vi "Main_RT.vi"() -> ()   [LabVIEW 2015]
uses:
  <vilib>/NI/Software Watchdog/Pound/Pound.lvclass
  <vilib>/addons/InsightCM/Devices/Shared/AcquireScanEngine/ScanEngine.lvlib
  <vilib>/addons/InsightCM/Devices/Shared/VibrationAnalysisLoop/VibrationAnalysis.lvlib
  <vilib>/addons/InsightCM/Devices/Shared/Trigger/Trigger.lvlib
  <vilib>/addons/InsightCM/Devices/Shared/TdmsCreator/TdmsCreator.lvlib
  <vilib>/addons/TraceLogger/TraceLogger.lvlib
  <vilib>/addons/TimerProcess/TimerProcess.lvlib
  <vilib>/addons/BlinkProcess/BlinkProcess.lvlib
  <vilib>/addons/InsightCM/Devices/Shared/Controller/Controller.lvlib
  <vilib>/addons/InsightCM/Devices/Shared/ServerComm/ServerComm.lvlib
  <vilib>/addons/InsightCM/Devices/Shared/FileManager/FileManager.lvlib
  <vilib>/addons/InsightCM/Devices/Shared/TracePointDisplay/TracePointDisplay.lvlib
  <vilib>/addons/InsightCM/Devices/Shared/TagPublish/TagPublish.lvlib
  <vilib>/addons/InsightCM/Devices/Shared/DataAccumulatorProcess/DataAccumulator.lvlib
  <vilib>/addons/InsightCM/Devices/Shared/DeviceHealth/DeviceHealth.lvlib
  <vilib>/addons/InsightCM/Devices/Shared/SinglePointClock/SinglePointClock.lvlib
  <vilib>/addons/InsightCM/Devices/Shared/VibrationVirtualChannel/VibrationVirtualChannel.lvlib
  <vilib>/addons/InsightCM/Devices/Shared/Alarm/Alarm.lvlib
  <vilib>/addons/InsightCM/Devices/Shared/TestPanel/TestPanel.lvlib
  <vilib>/addons/InsightCM/Devices/Shared/DataExplorerHelper/DataExplorerHelper.lvlib
  <vilib>/addons/InsightCM/Devices/Shared/ModbusMaster/ModbusMaster.lvlib
  <vilib>/addons/WatchdogProcess/WatchdogProcess.lvlib
panel:
  out "debug":string
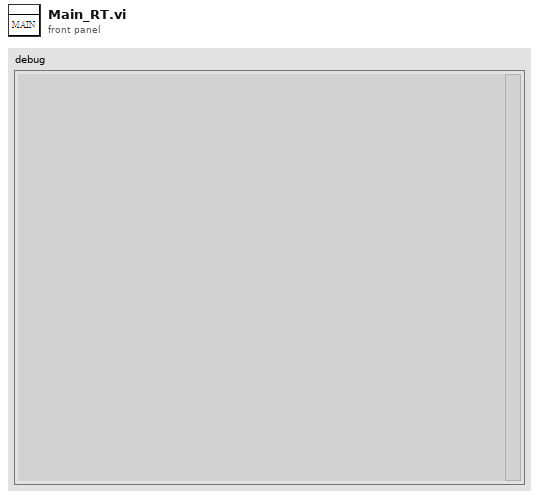
[diagram p1: front panel]
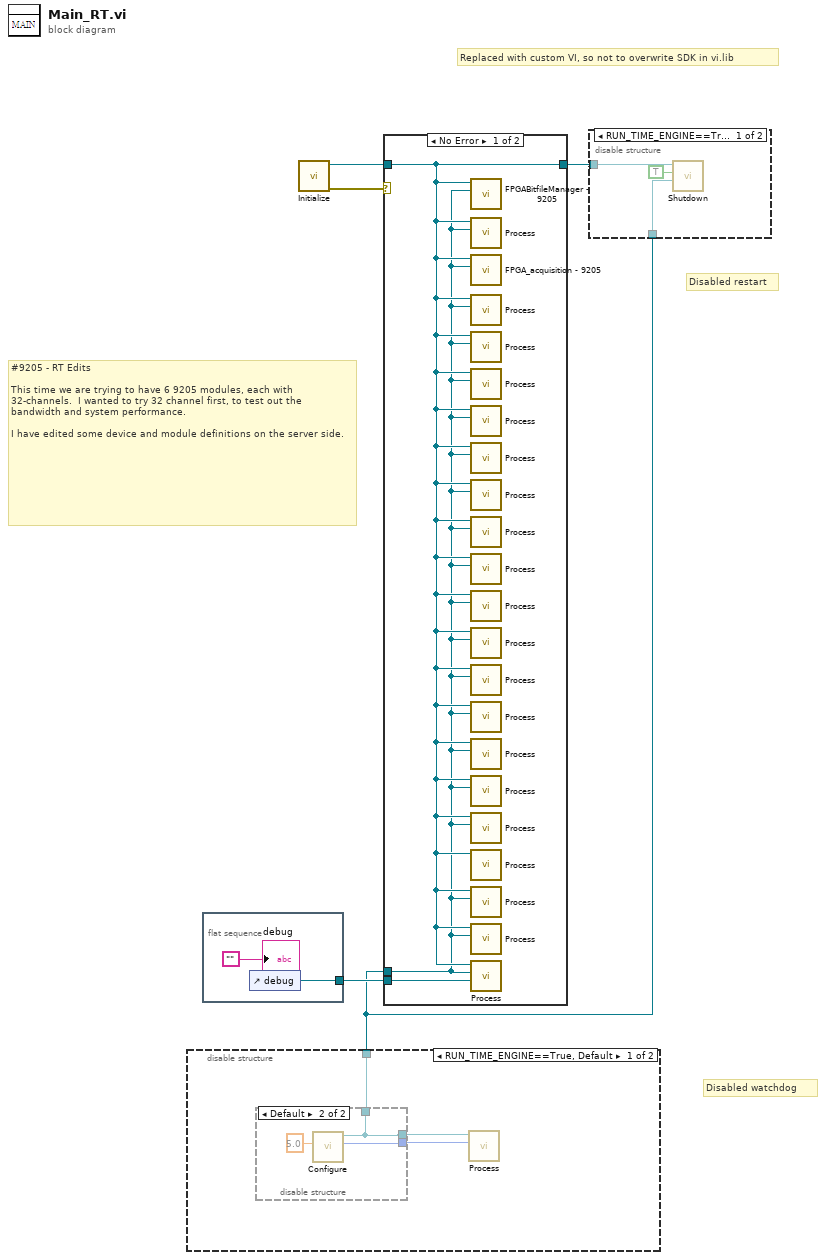
[diagram p0: block diagram]
diagram:
  # "Disabled watchdog"
  # "Disabled restart"
  # "Replaced with custom VI, so not to overwrite SDK in vi.lib"
  # "#9205 - RT Edits\n\nThis time we are trying to have 6 9205 modules, each with 32-channels.  I wanted to try 32 channel first, to test out the bandwidth and system performance.\n  \nI have edited some device and module definitions on the server side."
  n1 = disable-structure shown="RUN_TIME_ENGINE==True, Default" {
    disable-tunnel: [w8 _] -> w1
    frame condition #0 {
      n2 = disable-structure shown="Default" {
        disable-tunnel: [_ w10] -> w8
        disable-tunnel: [_ w10] -> w7
        disable-tunnel: [_ w9] -> w6
        frame condition #0 {
        }
        frame condition #1 (active) {
          n3 = call <vilib>:"Configure.vi"("hw timeout (sec)"=5.0) -> ("watchdogID out"=w9:u64, "Pound"=w10:refnum<class "Pound.lvclass">)  [unwired: 8 in, 1 out]
        }
      }
      n4 = call <vilib>:"Process.vi"("watchdogID"=w6, "Pound"=w7) -> ()  [unwired: 7 in, 3 out]
    }
    frame condition #1 (active) {
    }
  }
  n5 = flat-sequence {
    tunnel: [w12] -> w3
    frame #0 {
      n6 = control-ref of="debug"() -> (w12:refnum<vi>)
      "debug" <- ""
    }
  }
  n7 = call <vilib>:"Initialize.vi"() -> ("error out"=w5:errorcluster, "Qbus out"=w2:refnum<class "Qbus.lvclass">)  [unwired: 10 in]
  n8 = case shown="No Error" w5 {
    tunnel: w2 -> [w15 w17]
    tunnel: [w15 w17] -> w4
    tunnel: w1 -> [w14 _]
    tunnel: w3 -> [w16 _]
    frame No Error {
      n9 = call "FPGABitfileManager - 9205.vi"("Pound in"=w14, "Qbus in"=w15) -> ()  [unwired: 9 in, 1 out]
      n10 = call <vilib>:"Process.vi"("Pound in"=w14, "Qbus in"=w15) -> ()  [unwired: 9 in, 1 out]
      n11 = call "FPGA_acquisition - 9205.vi"("pound in"=w14, "qbus in"=w15) -> ()  [unwired: 9 in, 1 out]
      n12 = call <vilib>:"Process.vi"("Pound in"=w14, "Qbus in"=w15) -> ()  [unwired: 9 in, 1 out]
      n13 = call <vilib>:"Process.vi"("pound in"=w14, "qbus in"=w15) -> ()  [unwired: 9 in, 1 out]
      n14 = call <vilib>:"Process.vi"("Pound in"=w14, "Qbus in"=w15) -> ()  [unwired: 9 in, 1 out]
      n15 = call <vilib>:"Process.vi"("pound in"=w14, "Qbus in"=w15) -> ()  [unwired: 9 in, 1 out]
      n16 = call <vilib>:"Process.vi"("Pound in"=w14, "Qbus in"=w15) -> ()  [unwired: 9 in, 1 out]
      n17 = call <vilib>:"Process.vi"("Pound in"=w14, "Qbus in"=w15) -> ()  [unwired: 9 in, 1 out]
      n18 = call <vilib>:"Process.vi"("Pound in"=w14, "Qbus in"=w15) -> ()  [unwired: 9 in, 1 out]
      n19 = call <vilib>:"Process.vi"("Pound in"=w14, "Qbus in"=w15) -> ()  [unwired: 9 in, 1 out]
      n20 = call <vilib>:"Process.vi"("Pound in"=w14, "Qbus in"=w15) -> ()  [unwired: 9 in, 1 out]
      n21 = call <vilib>:"Process.vi"("Pound in"=w14, "Qbus in"=w15) -> ()  [unwired: 9 in, 1 out]
      n22 = call <vilib>:"Process.vi"("Pound in"=w14, "Qbus in"=w15) -> ()  [unwired: 9 in, 1 out]
      n23 = call <vilib>:"Process.vi"("Pound in"=w14, "Qbus in"=w15) -> ()  [unwired: 9 in, 1 out]
      n24 = call <vilib>:"Process.vi"("Pound in"=w14, "Qbus in"=w15) -> ()  [unwired: 9 in, 1 out]
      n25 = call <vilib>:"Process.vi"("Pound in"=w14, "Qbus in"=w15) -> ()  [unwired: 9 in, 1 out]
      n26 = call <vilib>:"Process.vi"("Pound in"=w14, "Qbus in"=w15) -> ()  [unwired: 9 in, 1 out]
      n27 = call <vilib>:"Process.vi"("qbus in"=w15) -> ()  [unwired: 10 in, 1 out]
      n28 = call <vilib>:"Process.vi"("Pound"=w14, "Qbus in"=w15) -> ()  [unwired: 9 in, 1 out]
      n29 = call <vilib>:"Process.vi"("pound in"=w14, "qbus in"=w15) -> ()  [unwired: 9 in, 1 out]
      n30 = call <vilib>:"Process.vi"("string refnum"=w16, "Pound in"=w14, "Qbus in"=w15) -> ()  [unwired: 8 in, 1 out]
    }
    frame Error {
    }
  }
  n31 = disable-structure shown="RUN_TIME_ENGINE==True, Default" {
    disable-tunnel: w4 -> [w20 _]
    disable-tunnel: w1 -> [w19 _]
    frame condition #0 {
      n32 = call <vilib>:"Shutdown.vi"("Pound"=w19, "restart system"=TRUE, "Qbus in"=w20) -> ()  [unwired: 8 in, 1 out]
    }
    frame condition #1 (active) {
    }
  }
